vi "Utility Error Query.vi"(5 "Retry Attempts (0)":i32 min=0, 8 "error in (no error)":errorcluster, 11 "VISA resource name":refnum<visa-resource-name>) -> (0 "error out":errorcluster, 1 "Error Message":string, 2 "Error Code":i32[](array[numeric]), 3 "VISA resource name out":refnum<visa-resource-name>)   [LabVIEW 2018, in "ChromTech MX-Class Drivers.lvlib"]
doc: "Queries the instrument for any errors in the instrument's error queue. It will continue to read errors until all errors have been read from the instrument. Any errors will be returned in the <B>error out</B> control.\n\n<B>Note:</B>\nThis VI is called automatically by most driver VIs so it is not usually necessary to call this in an application."
uses:
  <instrlib>/ChromTech MX-Class Pump/ChromTech MX-Class Drivers.lvlib
panel:
  # "EDIT: Note: The Error Query VI is included as a subVI in all driver VIs except low-level API VIs. If the instrument does not support error query, then remove the VI and remove subVI calls in each instrument driver VI that calls it."
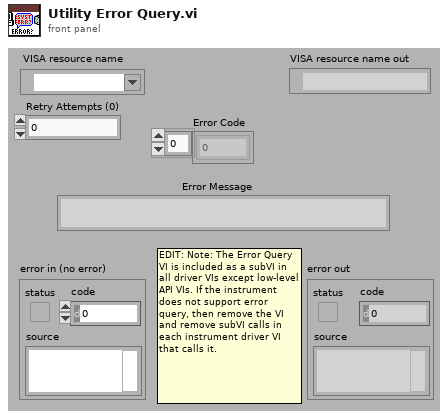
[diagram p1: front panel]
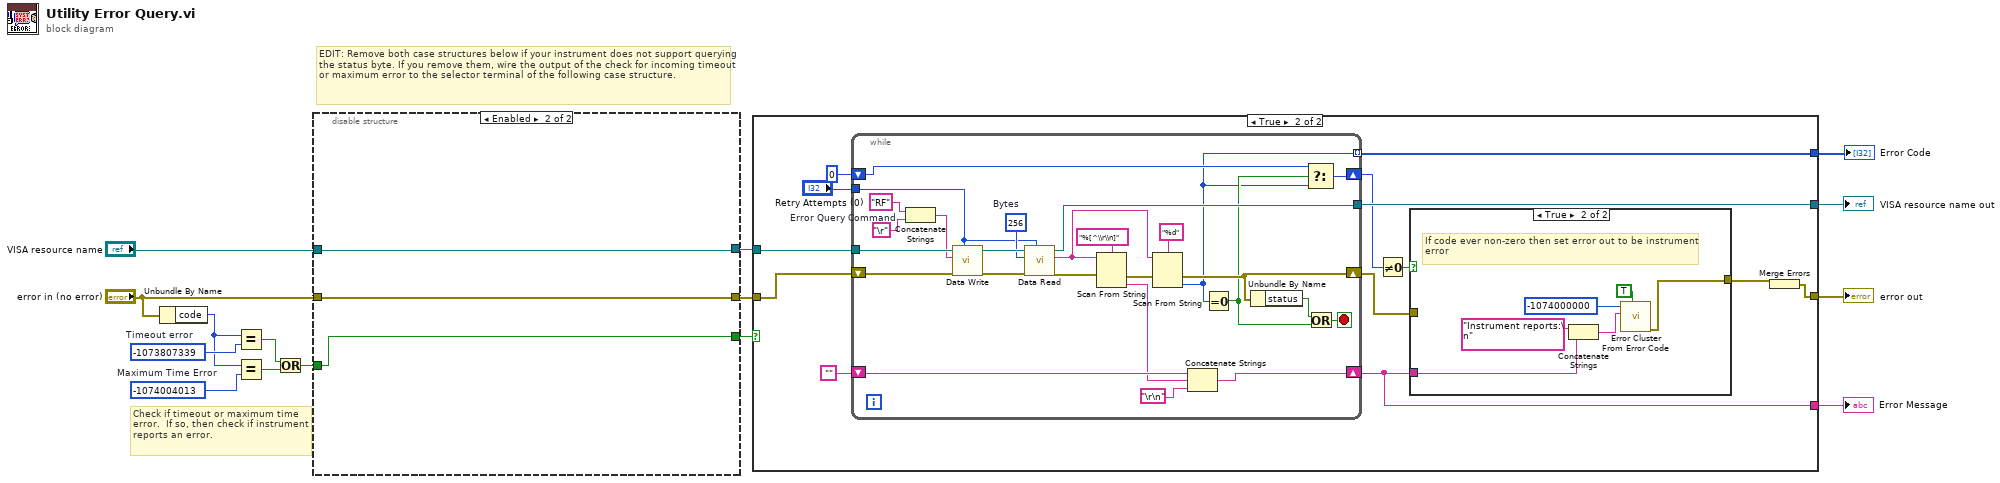
[diagram p0: block diagram]
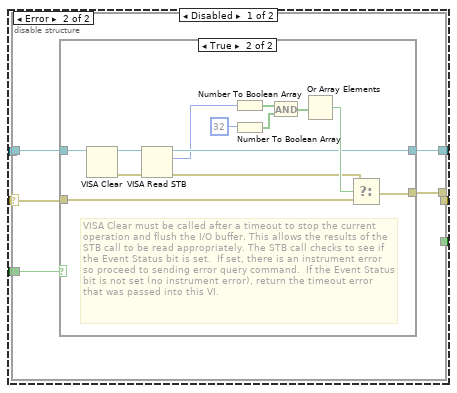
[diagram p2: hidden frame]
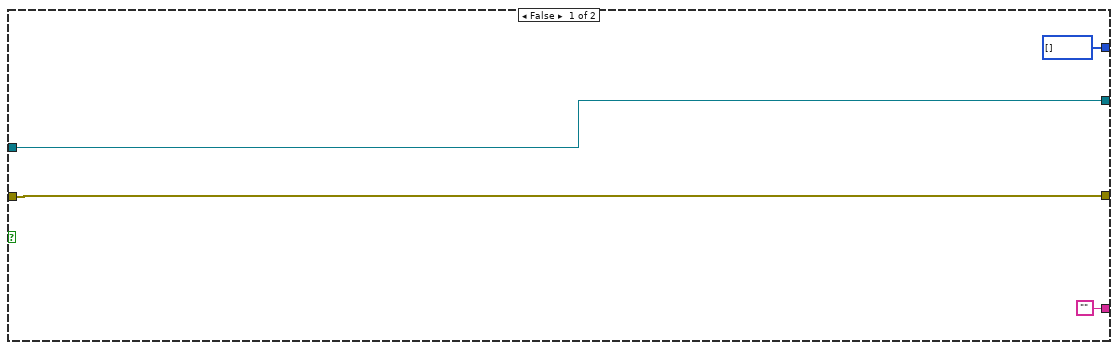
[diagram p5: hidden frame]
diagram:
  w7 = -1074004013  # Maximum Time Error
  w9 = -1073807339  # Timeout error
  # "Check if timeout or maximum time error.  If so, then check if instrument reports an error."
  # "EDIT: Remove both case structures below if your instrument does not support querying the status byte. If you remove them, wire the output of the check for incoming timeout or maximum error to the selector terminal of the following case structure."
  n1 = Unbundle By Name("error in (no error)") -> ("code"=w8:i32)
  n2 = Equal?(x=w8, y=w9) -> (x = y?=w5:bool)
  n3 = Equal?(x=w8, y=w7) -> (x = y?=w6:bool)
  n4 = Or(x=w5, y=w6) -> (x .or. y?=w4:bool)
  n5 = disable-structure shown="Enabled" {
    disable-tunnel: [w20 w45] -> w2
    disable-tunnel: [w19 w44] -> w11
    disable-tunnel: "VISA resource name" -> [w18 w44]
    disable-tunnel: w4 -> [w17 w43]
    disable-tunnel: "error in (no error)" -> [w16 w45]
    disable-tunnel: [_ w43] -> w1
    frame Disabled {
      n6 = case shown="Error" w16 {
        selector: w16 -> [w21 w25]
        tunnel: w18 -> [w22 w27]
        tunnel: [w22 w26] -> w19
        tunnel: [w21 w24] -> w20
        tunnel: w17 -> [_ w23]
        frame No Error {
        }
        frame Error {
          n7 = case shown="True" w23 {
            tunnel: w27 -> [w29 w35]
            tunnel: [w29 w32] -> w26
            tunnel: w25 -> [w28 w38]
            tunnel: [w28 w37] -> w24
            frame False {
              # "Error code not a timeout, so best to pass on to user."
            }
            frame True {
              # "VISA Clear must be called after a timeout to stop the current operation and flush the I/O buffer. This allows the results of the  STB call to be read appropriately. The STB call checks to see if the Event Status bit is set.  If set, there is an instrument error so proceed to sending error query command.  If the Event Status bit is not set (no instrument error), return the timeout error that was passed into this VI."
              n8 = VISA Clear(VISA resource name=w35) -> (VISA resource name out=w34:refnum<visa-resource-name>, error out=w33:errorcluster)  [unwired: 1 in]
              n9 = VISA Read STB(8:w33, 11:w34) -> (0:w31:errorcluster, 2:w30:u16, 3:w32:refnum<visa-resource-name>)
              n10 = Number To Boolean Array(number=w30) -> (Boolean array=w39:bool[])
              n11 = Number To Boolean Array(number=32) -> (Boolean array=w41:bool[])
              n12 = And(x=w39, y=w41) -> (x .and. y?=w40:bool[])
              n13 = Or Array Elements(Boolean array=w40) -> (logical OR=w36:bool)
              n14 = Select(t=w31, s=w36, f=w38) -> (s? t:f=w37:errorcluster)
            }
          }
        }
      }
    }
    frame Enabled {
    }
  }
  n15 = case shown="True" w1 {
    tunnel: [w49 w62] -> w15
    tunnel: w11 -> [w49 w61]
    tunnel: [w46 w59] -> w14
    tunnel: ["" w54] -> w13
    tunnel: [i32[] [] w53] -> w12
    tunnel: w2 -> [w46 w51]
    frame False {
    }
    frame True {
      n16 = while {
        tunnel: [w95] -> w62
        tunnel: w61 -> [w94]
        shift-right: [w83] -> w54
        shift-left: "" -> [w86]
        shift-right: [w81] -> w55
        shift-left: 0 -> [w82]
        shift-right: [w79] -> w52
        shift-left: w51 -> [w80]
        tunnel: [w74] -> w53 mode=indexing
        tunnel: "Retry Attempts (0)" -> [w70]
        stop <- w89 stop-if-true
        w92 = u32 256  # Bytes
        w72 = "RF"  # Error Query Command
        n17 = Concatenate Strings(w72, "\r") -> (w71:string)
        n18 = call <instrlib>:"Data Write.vi"("Retry Attempts (0)"=w70, "error in (no error)"=w80, "Command"=w71, "VISA Refnum in"=w94) -> ("error out"=w91:errorcluster, "VISA Refnum out"=w93:refnum<visa-resource-name>)  [unwired: 6 in]
        n19 = call <instrlib>:"Data Read.vi"("Retry Attempts (0)"=w70, "error in (no error)"=w91, "Bytes to read"=w92, "VISA Refnum in"=w93) -> ("error out"=w78:errorcluster, "read buffer"=w87:string, "VISA Refnum out"=w95:refnum<visa-resource-name>)  [unwired: 5 in]
        n20 = Scan From String(format string="%[^\\r\\n]", input string=w87, error in=w78) -> (error out=w77:errorcluster, output 1=w84:string)  [unwired: 2 in, 2 out]
        n21 = Scan From String(format string="%d", input string=w87, error in=w77) -> (error out=w79:errorcluster, output 1=w74:i32)  [unwired: 2 in, 2 out]
        n22 = Concatenate Strings(w86, w84, "\r\n") -> (w83:string)
        n23 = Equal To 0?(x=w74) -> (x = 0?=w75:bool)
        n24 = Unbundle By Name(w79) -> ("status"=w76:bool)
        n25 = Select(t=w82, s=w75, f=w74) -> (s? t:f=w81:i32)
        n26 = Or(x=w76, y=w75) -> (x .or. y?=w89:bool)
      }
      n27 = Not Equal To 0?(x=w55) -> (x != 0?=w57:bool)
      n28 = case shown="True" w57 {
        tunnel: w54 -> [_ w68]
        tunnel: [w63 w64] -> w56
        tunnel: w52 -> [w63 _]
        frame False {
        }
        frame True {
          # "If code ever non-zero then set error out to be instrument error"
          n29 = Concatenate Strings("Instrument reports:\n" ("Source"), w68) -> (w65:string)
          n30 = call <vilib>:"Error Cluster From Error Code.vi"("show call chain? (False)"=TRUE, "error message (\"\")"=w65, "error code (0)"=-1074000000 ("Code")) -> ("error out"=w64:errorcluster)  [unwired: 6 in]
        }
      }
      n31 = Merge Errors(w56) -> (w59:errorcluster)
    }
  }
  "VISA resource name out" <- w15
  "error out" <- w14
  "Error Message" <- w13
  "Error Code" <- w12
